vi "Query Filter.vi"(8 "error in (no error)":errorcluster, 11 "VISA resource name":refnum<visa-resource-name>) -> (0 "error out":errorcluster, 2 "CURRENT FILTER":u8 step=2, 3 "VISA resource name out":refnum<visa-resource-name>)   [LabVIEW 2017, in "Digikrom DK24x.lvlib"]
doc: "Returns the current filter setting."
uses:
  Digikrom DK24x.lvlib
  Private/Filter State.vi
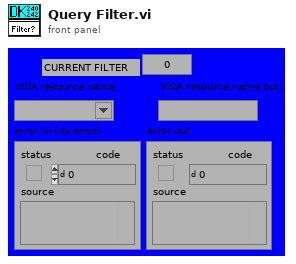
[diagram p1: front panel]
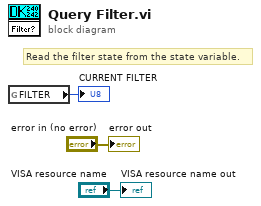
[diagram p0: block diagram]
diagram:
  # "Read the filter state from the state variable."
  n1 = global read "Filter State.vi" "FILTER"() -> (→"CURRENT FILTER":u8)
  "error out" <- "error in (no error)"
  "VISA resource name out" <- "VISA resource name"
